vi "Main Page.vi"(8 "error in (no error)":errorcluster, 11 "Node Ptr":T1 format="%.0x") -> (0 "error out":errorcluster)   [LabVIEW 2020, in "PXI-2514 System Explorer.lvlib"]
uses:
  PXI-2514 System Explorer.lvlib
  <vilib>/NI VeriStand/Custom Device API/Custom Device Item Ref.ctl
  <vilib>/NI VeriStand/Custom Device API/Set Item Property (U16).vi
  <vilib>/NI VeriStand/Custom Device API/Get Item Property (U16).vi
  <vilib>/NI VeriStand/Custom Device API/Custom Device API.lvlib
  <vilib>/NI VeriStand/Custom Device API/Set Item Property (String).vi
  Shared/Constants.vi
  Shared/PXI-2514 Shared.lvlib
  <vilib>/NI VeriStand/Custom Device API/Get Item Property (String).vi
panel:
  in  "Hardware Device Name":string caption="This is the device name which appears \nin Measurement and Automation\n Explorer (MAX)"
  in  "Async Timeout (ms)":u16
  out "Version":string
  in  "General Header":cluster{"Section Name":string}={"Section Name"="General Custom Device Settings"}
  in  "Description":string
  in  "Name":string
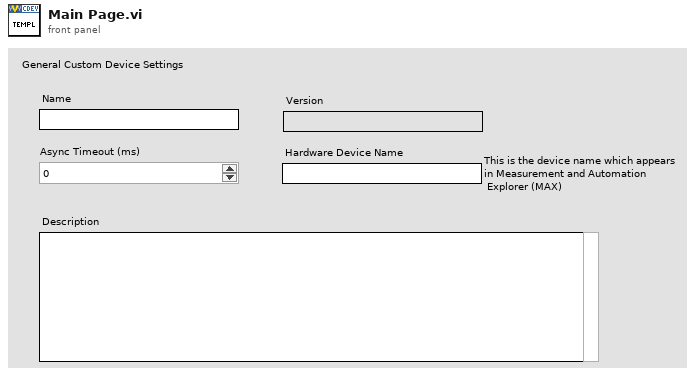
[diagram p1: front panel]
types:
  T1 = typedef "Custom Device API.lvlib/Custom Device Item Ref.ctl" = u64
  T2 = typedef "Custom Device API.lvlib/Custom Device Item Info.ctl" = cluster{"Name":string, "Is Channel":bool, "GUID":string, "Is Waveform":bool}
  T3 = typedef "Custom Device API.lvlib/Custom Device Commands.ctl" = enum16{"Default", "Item renamed", "Shutdown", "Dynamic button pressed"}
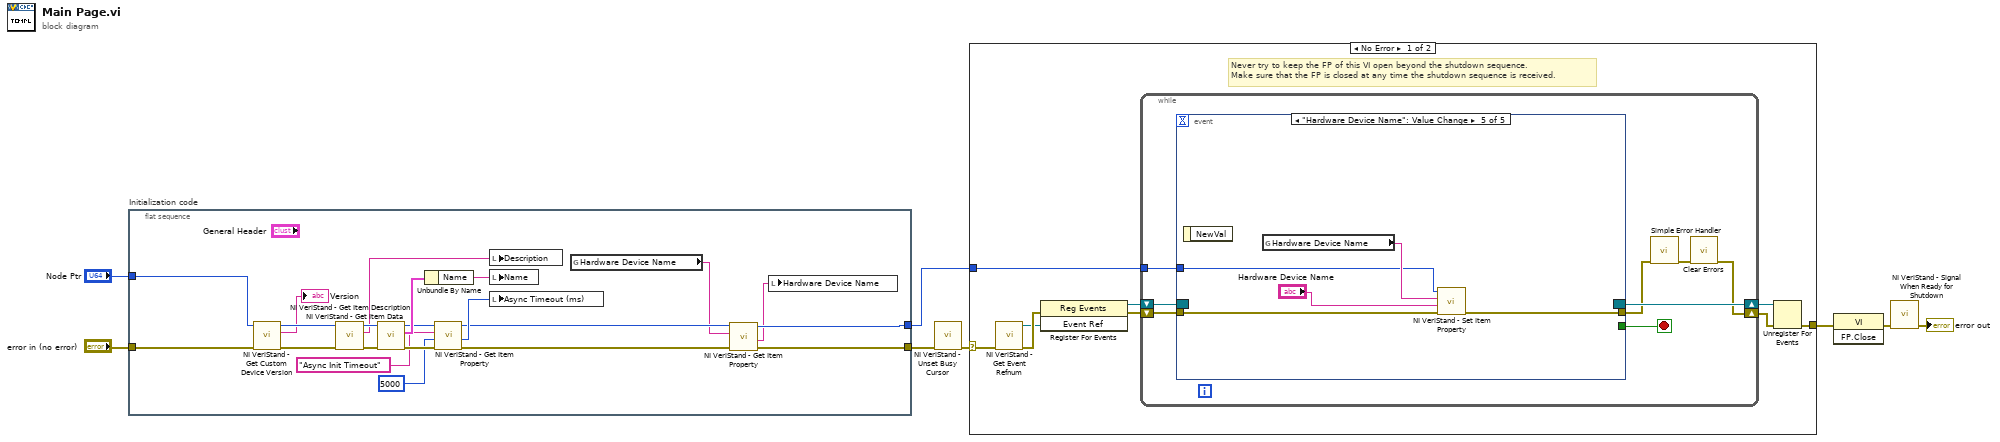
[diagram p0: block diagram]
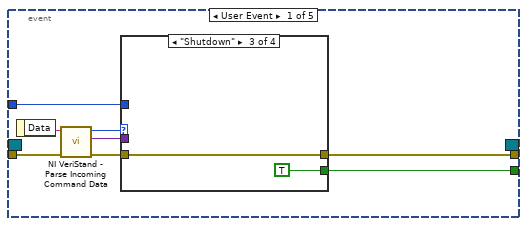
[diagram p2: hidden frame]
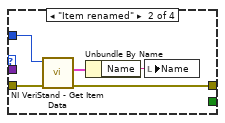
[diagram p4: hidden frame]
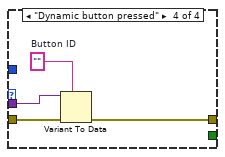
[diagram p5: hidden frame]
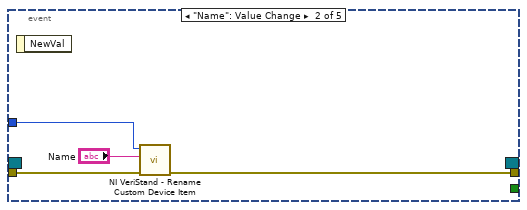
[diagram p6: hidden frame]
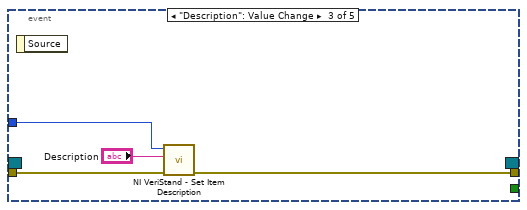
[diagram p7: hidden frame]
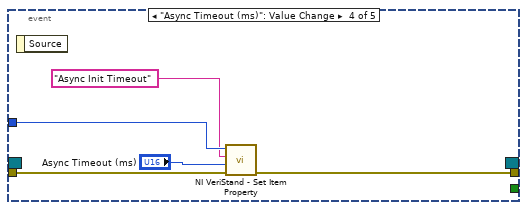
[diagram p8: hidden frame]
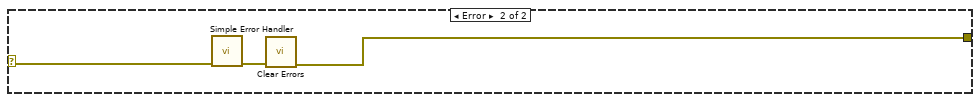
[diagram p9: hidden frame]
diagram:
  n1 = flat-sequence "Initialization code" {
    tunnel: "error in (no error)" -> [w15]
    tunnel: "Node Ptr" -> [w26]
    tunnel: [w14] -> w4
    tunnel: [w13] -> w1
    frame #0 {
      n2 = call <vilib>:"NI VeriStand - Get Custom Device Version.vi"("error in (no error)"=w15, "Device Ref in"=w26) -> ("error out"=w25:errorcluster, "Value"=→"Version":string, "Device Ref out"=w24:T1)  [unwired: 7 in]
      n3 = call <vilib>:"NI VeriStand - Get Item Description.vi"("error in (no error)"=w25, "Item Ref in"=w24) -> ("error out"=w28:errorcluster, "Description"=w21:string, "Item Ref out"=w29:T1)  [unwired: 7 out]
      n4 = call <vilib>:"NI VeriStand - Get Item Data.vi"("error in (no error)"=w28, "Item Ref in"=w29) -> ("error out"=w20:errorcluster, "Item Info"=w27:T2, "Item Ref out"=w19:T1)  [unwired: 7 out]
      n5 = Unbundle By Name(w27) -> ("Name"=w22:string)
      n6 = call-poly <vilib>:"NI VeriStand - Get Item Property.vi"("error in (no error)"=w20, "Default Value"=u16 5000, "Property Name"="Async Init Timeout", "Item Ref in"=w19) -> ("error out"=w11:errorcluster, "Value"=w18:u16, "Item Ref out"=w12:T1)  [unwired: 4 in, 1 out]
      n7 = local write "Description"(w21) -> ()
      n8 = local write "Name"(w22) -> ()
      n9 = local write "Async Timeout (ms)"(w18) -> ()
      n10 = global read "Constants.vi" "Hardware Device Name"() -> (w9:string)
      n11 = call-poly <vilib>:"NI VeriStand - Get Item Property.vi"("error in (no error)"=w11, "Property Name"=w9, "Item Ref in"=w12) -> ("error out"=w14:errorcluster, "Value"=w10:string, "Item Ref out"=w13:T1)  [unwired: 5 in, 1 out]
      n12 = local write "Hardware Device Name"(w10) -> ()
    }
  }
  n13 = call <vilib>:"NI VeriStand - Unset Busy Cursor.vi"("error in (no error)"=w4) -> ("error out"=w3:errorcluster)  [unwired: 10 out]
  n14 = case shown="No Error" w3 {
    selector: w3 -> [w30 w87]
    tunnel: [w35 w85] -> w8
    tunnel: w1 -> [w31 _]
    frame No Error {
      # "Never try to keep the FP of this VI open beyond the shutdown sequence.\nMake sure that the FP is closed at any time the shutdown sequence is received."
      n15 = call <vilib>:"NI VeriStand - Get Event Refnum.vi"("error in (no error)"=w30) -> ("error out"=w38:errorcluster, "Event Ref"=w34:refnum<user-event>)  [unwired: 9 out]
      n16 = register-events(error in=w38, w34) -> (reference out=w32:refnum<event-registration>, error out=w33:errorcluster)  [unwired: 1 in]
      n17 = while {
        tunnel: w31 -> [w42]
        shift-right: [w39] -> w36
        shift-left: w33 -> [w45]
        shift-right: [w46] -> w37
        shift-left: w32 -> [w44]
        stop <- w43 stop-if-true
        n18 = event shown="[4] \"Hardware Device Name\": Value Change" {
          selector: w44 -> [_ _ _ _ _]
          dyn-events: [_ _ _ _ _] -> w46
          timeout: _ -> [_ _ _ _ _]
          tunnel: w45 -> [w54 w70 w73 w79 w84]
          tunnel: [w50 _ _ _ _] -> w43
          tunnel: [w49 w69 w72 w76 w83] -> w41
          tunnel: w42 -> [w48 w68 w74 w78 w80]
          event User Event {
            n19 = event-data() -> ("Data"=w53:string)  [unwired: 1 out]
            n20 = call <vilib>:"NI VeriStand - Parse Incoming Command Data.vi"("error in (no error)"=w54, "Incoming data"=w53) -> ("error out"=w52:errorcluster, "Outgoing data"=w47:variant, "Action"=w51:T3)  [unwired: 7 out]
            n21 = case shown="\"Shutdown\"" w51 {
              tunnel: w52 -> [w55 w60 w61 w66]
              tunnel: [_ _ TRUE _] -> w50
              tunnel: [w55 w57 w61 w63] -> w49
              tunnel: w48 -> [_ w59 _ _]
              tunnel: w47 -> [_ _ _ w65]
              frame "Default", Default {
              }
              frame "Item renamed" {
                n22 = call <vilib>:"NI VeriStand - Get Item Data.vi"("error in (no error)"=w60, "Item Ref in"=w59) -> ("error out"=w57:errorcluster, "Item Info"=w58:T2)  [unwired: 8 out]
                n23 = Unbundle By Name(w58) -> ("Name"=w56:string)
                n24 = local write "Name"(w56) -> ()
              }
              frame "Shutdown" {
              }
              frame "Dynamic button pressed" {
                w64 = ""  # Button ID
                n25 = Variant To Data(error in=w66, type=w64, Variant=w65) -> (error out=w63:errorcluster)  [unwired: 1 out]
              }
            }
          }
          event "Name": Value Change {
            n26 = event-data() -> ()  [unwired: 2 out]
            n27 = call <vilib>:"NI VeriStand - Rename Custom Device Item.vi"("error in (no error)"=w70, "New Name"="Name", "Item Ref in"=w68) -> ("error out"=w69:errorcluster)  [unwired: 1 in, 7 out]
          }
          event "Description": Value Change {
            n28 = event-data() -> ()  [unwired: 2 out]
            n29 = call <vilib>:"NI VeriStand - Set Item Description.vi"("error in (no error)"=w73, "Description"="Description", "Item Ref in"=w74) -> ("error out"=w72:errorcluster)  [unwired: 8 out]
          }
          event "Async Timeout (ms)": Value Change {
            n30 = event-data() -> ()  [unwired: 2 out]
            n31 = call-poly <vilib>:"NI VeriStand - Set Item Property.vi"("error in (no error)"=w79, "Value"="Async Timeout (ms)", "Property Name"="Async Init Timeout", "Item Ref in"=w78) -> ("error out"=w76:errorcluster)  [unwired: 5 in, 2 out]
          }
          event "Hardware Device Name": Value Change {
            n32 = event-data() -> ()  [unwired: 2 out]
            n33 = global read "Constants.vi" "Hardware Device Name"() -> (w82:string)
            n34 = call-poly <vilib>:"NI VeriStand - Set Item Property.vi"("error in (no error)"=w84, "Value"="Hardware Device Name", "Property Name"=w82, "Item Ref in"=w80) -> ("error out"=w83:errorcluster)  [unwired: 5 in, 2 out]
          }
        }
        n35 = call <vilib>:"Simple Error Handler.vi"("error in (no error)"=w41) -> ("error out"=w40:errorcluster)  [unwired: 1 in, 7 out]
        n36 = call <vilib>:"Clear Errors.vi"("error in (no error)"=w40) -> ("error out"=w39:errorcluster)  [unwired: 1 in, 5 out]
      }
      n37 = Unregister For Events(event registration refnum=w37, error in=w36) -> (error out=w35:errorcluster)
    }
    frame Error {
      n38 = call <vilib>:"Simple Error Handler.vi"("error in (no error)"=w87) -> ("error out"=w86:errorcluster)  [unwired: 1 in, 7 out]
      n39 = call <vilib>:"Clear Errors.vi"("error in (no error)"=w86) -> ("error out"=w85:errorcluster)  [unwired: 1 in, 5 out]
    }
  }
  n40 = invoke class="VI" method="FP.Close"(error in=w8) -> (error out=w7:errorcluster)  [unwired: 2 in, 2 out]
  n41 = call <vilib>:"NI VeriStand - Signal When Ready for Shutdown.vi"("error in (no error)"=w7) -> ("error out"=→"error out":errorcluster)  [unwired: 10 out]
